vi "Set_Get_Path_DLL.vi"(10 "Add Path DLL (False)":bool, 11 "path DLL":path) -> (3 "path DLL Out":path)   [LabVIEW 2018]
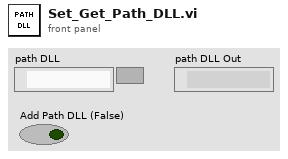
[diagram p1: front panel]
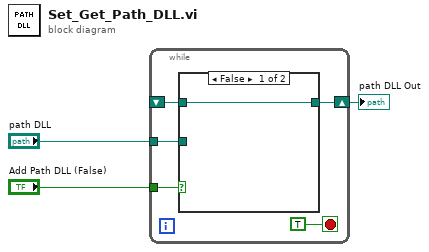
[diagram p0: block diagram]
diagram:
  n1 = while {
    tunnel: "Add Path DLL (False)" -> [w7]
    shift-right: [w6] -> w3
    shift-left: _ -> [w4]
    tunnel: "path DLL" -> [w5]
    stop <- TRUE stop-if-true
    n2 = case shown="False" w7 {
      tunnel: [w9 w10] -> w6
      tunnel: w5 -> [_ w10]
      tunnel: w4 -> [w9 _]
      frame False {
      }
      frame True {
      }
    }
  }
  "path DLL Out" <- w3
